vi "read includes file path.vi"(8 "error in":errorcluster, 11 "Targets in":refnum<class "Targets.lvclass">) -> (0 "error out":errorcluster, 2 "Path":path, 3 "Targets out":refnum<class "Targets.lvclass">)   [LabVIEW 2013, in "PL Framework Configuration Tool.lvlib" / "Targets.lvclass"]
uses:
  Targets.lvclass
  <vilib>/NI/Configuration Framework/serializable configuration/NISE_CEF_serializable configuration.lvclass
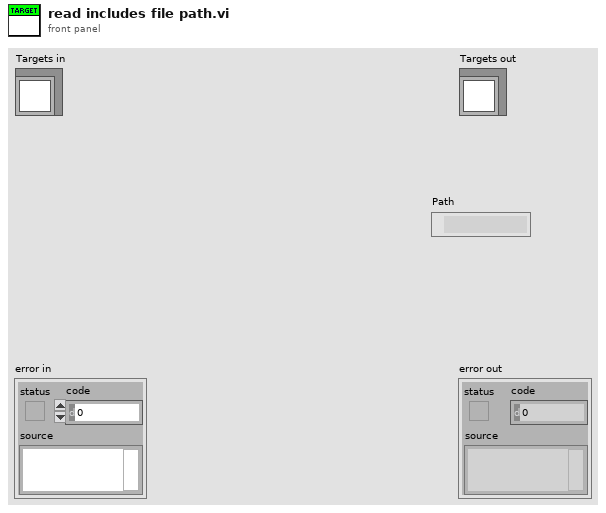
[diagram p1: front panel]
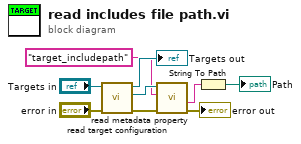
[diagram p0: block diagram]
diagram:
  n1 = call "read target configuration.vi"("error in"="error in", "Targets in"="Targets in") -> ("error out"=w6:errorcluster, "Target Configuration"=w4:refnum<class "PL_Target Configuration.lvclass">, "Targets out"=→"Targets out":refnum<class "Targets.lvclass">)  [unwired: 7 in]
  n2 = call <vilib>:"read metadata property.vi"("error in"=w6, "key"="target_includepath", "configuration in"=w4) -> ("error out"=→"error out":errorcluster, "value"=w1:string)  [unwired: 5 in, 2 out]
  n3 = String To Path(string=w1) -> (path=→"Path":path)
